vi "Table.vi"() -> ()   [LabVIEW 2012]
uses:
  Controls/TestData.ctl
  <vilib>/Utility/file.llb/Write To Spreadsheet File (string).vi
panel:
  out "Array":string[](array[string])
  in  "file path (dialog if empty)":path
  out "Table":string[][](table)
  in  "TestData":T1 {"50mA Data"."Current,mA" format="%_6g"; "50mA Data"."WL" format="%_6g"; "50mA Data"."Voltage" format="%_6g"; "50mA Data"."Power" format="%_6g"; "20mA Data"."Reverse" format="%#_3g"; "20mA Data"."Current,mA" format="%_6g"; "20mA Data"."Knee Current" format="%#_3g"; "20mA Data"."WL" format="%_6g"; "20mA Data"."Voltage" format="%_6g"; "20mA Data"."Power" format="%_5g"}
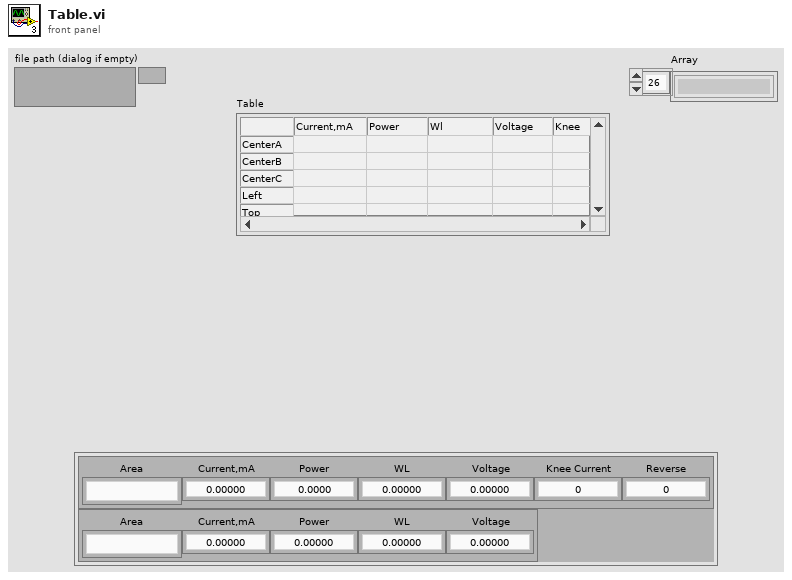
[diagram p1: front panel]
types:
  T1 = typedef "TestData.ctl" = cluster{"20mA Data":cluster{"Area":string, "Current,mA":dbl, "Power":dbl, "WL":dbl, "Voltage":dbl, "Knee Current":dbl, "Reverse":dbl}, "50mA Data":cluster{"Area":string, "Current,mA":dbl, "Power":dbl, "WL":dbl, "Voltage":dbl}}
  T2 = cluster{"Area":string, "Current,mA":dbl, "Power":dbl, "WL":dbl, "Voltage":dbl, "Knee Current":dbl, "Reverse":dbl}
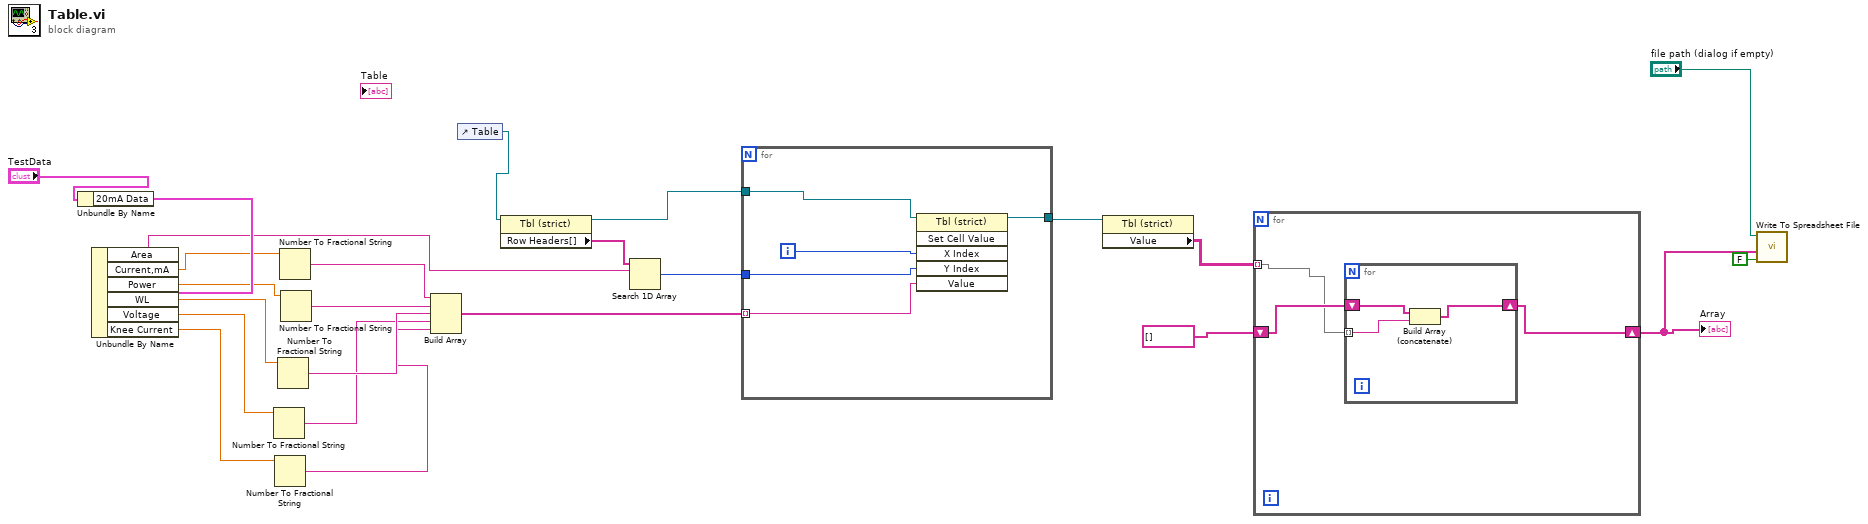
[diagram p0: block diagram]
diagram:
  n1 = Unbundle By Name("TestData") -> ("20mA Data"=w23:T2)
  n2 = Unbundle By Name(w23) -> ("Area"=w3:string, "Current,mA"=w2:dbl, "Power"=w22:dbl, "WL"=w21:dbl, "Voltage"=w20:dbl, "Knee Current"=w19:dbl)
  n3 = Number To Fractional String(number=w20) -> (F-format string=w16:string)  [unwired: 3 in]
  n4 = Number To Fractional String(number=w19) -> (F-format string=w15:string)  [unwired: 3 in]
  n5 = Number To Fractional String(number=w21) -> (F-format string=w17:string)  [unwired: 3 in]
  n6 = Number To Fractional String(number=w2) -> (F-format string=w1:string)  [unwired: 3 in]
  n7 = Number To Fractional String(number=w22) -> (F-format string=w18:string)  [unwired: 3 in]
  n8 = Build Array(w1, w18, w17, w16, w15) -> (w12:string[])
  n9 = control-ref of="Table"() -> (w11:refnum<vi>)
  n10 = property class="Tbl (strict)"(reference=w11) -> (reference out=w10:refnum<vi>, "Row Headers[]"=w14:string[])  [unwired: 1 in, 1 out]
  n11 = Search 1D Array(1D array=w14, element=w3) -> (index of element=w13:i32)  [unwired: 1 in]
  n12 = for {
    tunnel: w13 -> [w29]
    tunnel: w12 -> [w27] mode=indexing
    tunnel: w10 -> [w26]
    tunnel: [w25] -> w9
    i -> [w28]
    n13 = invoke class="Tbl (strict)" method="Set Cell Value"(reference=w26, "X Index"=w28, "Y Index"=w29, "Value"=w27) -> (reference out=w25:refnum<vi>)  [unwired: 2 in, 5 out]
  }
  n14 = property class="Tbl (strict)"(reference=w9) -> ("Value"=w5:string[][])  [unwired: 1 in, 2 out]
  n15 = for {
    tunnel: w5 -> [w31] mode=indexing
    shift-right: [w30] -> w4
    shift-left: string[] [] -> [w32]
    n16 = for {
      shift-right: [w33] -> w30
      shift-left: w32 -> [w35]
      tunnel: w31 -> [w34] mode=indexing
      n17 = Build Array (concatenate)(w35, w34) -> (w33:string[])
    }
  }
  "Array" <- w4
  n18 = call-poly <vilib>:"Write To Spreadsheet File.vi"("append to file? (new file:F)"=FALSE, "1D data"=w4, "file path (dialog if empty)"="file path (dialog if empty)") -> ()  [unwired: 5 in, 1 out]
